vi "Facade.vi"(0 "Data In":T6, 2 "Display State In":T2={"Prompt"="Click to add", "Listbox"=refnum, "Required"={"Strings"=[], "Bottom"=FALSE, "Italic"=FALSE, "FG"=0, "BG"=0, "Bold"=FALSE}, "Items"=[], "Req'd"=[], "Events"={"Items Changed"=refnum, "List Changed"=refnum}, "Max Rows"=-1, "Default name"=""}, 3 "Container State":T5) -> (6 "Data Out":T6, 7 "Display State Out":T2={"Prompt"="Click to add", "Listbox"=refnum, "Required"={"Strings"=[], "Bottom"=FALSE, "Italic"=FALSE, "FG"=0, "BG"=0, "Bold"=FALSE}, "Items"=[], "Req'd"=[], "Events"={"Items Changed"=refnum, "List Changed"=refnum}, "Max Rows"=-1, "Default name"=""}, 8 "Action":T1)   [LabVIEW 2015, in "KListboxEx.xctl"]
uses:
  KListboxEx.xctl
  Data.ctl
  <vilib>/_xctls/Container State.ctl
  State.ctl
  Required.ctl
  Events.ctl
  Event Action.ctl
  <vilib>/_xctls/Action.ctl
  <vilib>/_xctls/XControlSupport.lvlib
panel:
  out "redisplay":bool
  out "drag from":i32
  in  "Listbox":i32(listbox)
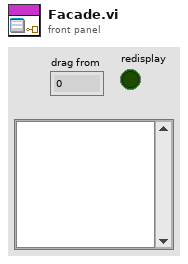
[diagram p1: front panel]
types:
  T1 = typedef "XControlSupport.lvlib/Action.ctl" = cluster{"Data Changed?":bool, "State Changed?":bool, "Action Name":string}
  T2 = typedef "KListboxEx.xctl/State.ctl" = cluster{"Prompt":string, "Listbox":refnum<vi>, "Required":T3, "Items":string[], "Req'd":bool[], "Events":T4, "Max Rows":i32, "Default name":string}
  T3 = typedef "KListboxEx.xctl/Required.ctl" = cluster{"Strings":string[], "Bottom":bool, "Italic":bool, "FG":u32, "BG":u32, "Bold":bool}
  T4 = typedef "KListboxEx.xctl/Events.ctl" = cluster{"Items Changed":refnum<user-event>, "List Changed":refnum<user-event>}
  T5 = typedef "XControlSupport.lvlib/Container State.ctl" = cluster{"Indicator?":bool, "Run Mode?":bool, " Refnum":refnum<vi>}
  T6 = typedef "KListboxEx.xctl/Data.ctl" = i32
  T7 = typedef "KListboxEx.xctl/Event Action.ctl" = enum16{"None", "Add", "Delete", "Move", "Edit", "Select"}
  T8 = typedef "LVPoint32TypeDef.ctl" = cluster{"Horizontal":i32, "Vertical":i32}
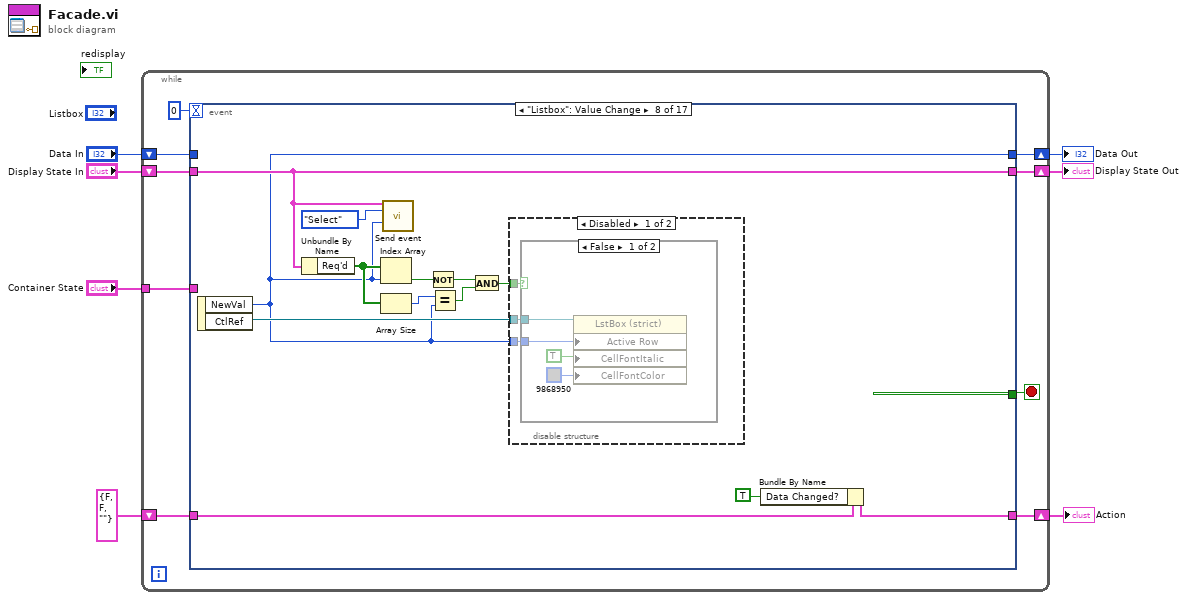
[diagram p0: block diagram]
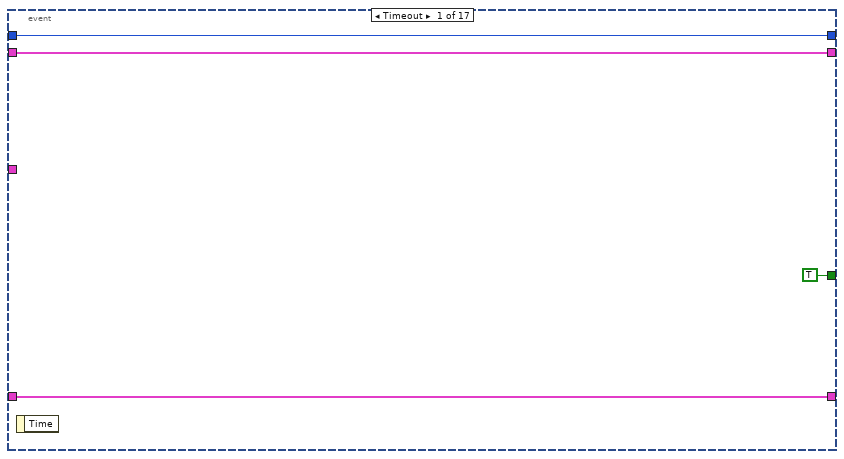
[diagram p2: hidden frame]
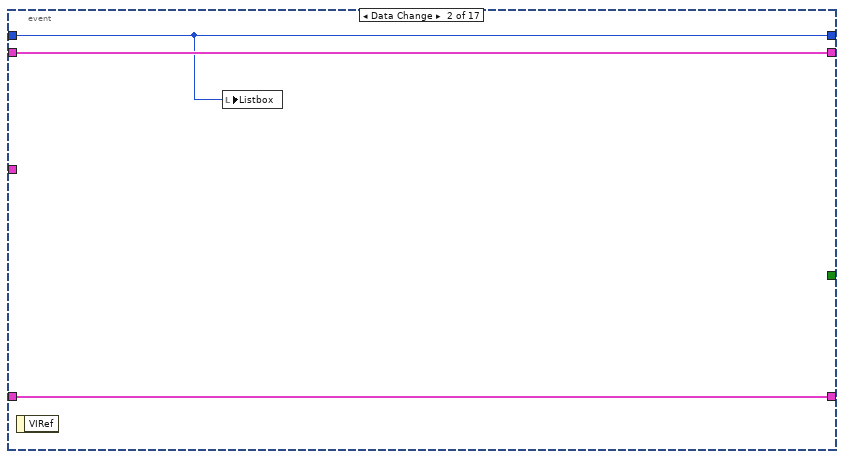
[diagram p3: hidden frame]
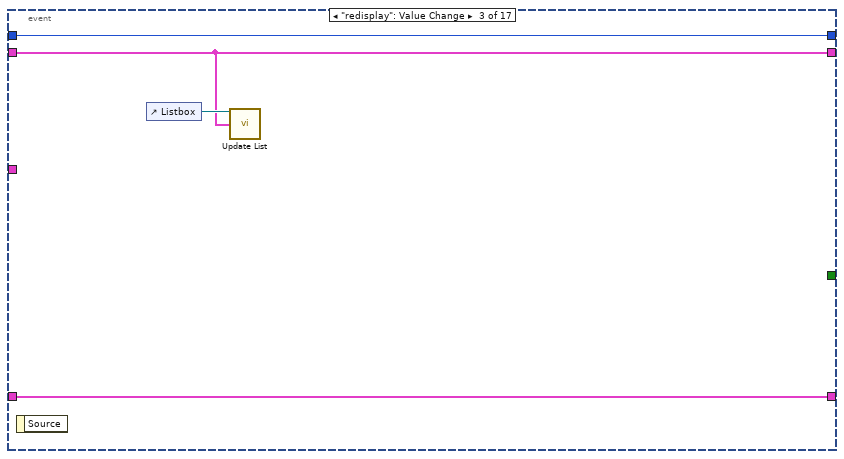
[diagram p4: hidden frame]
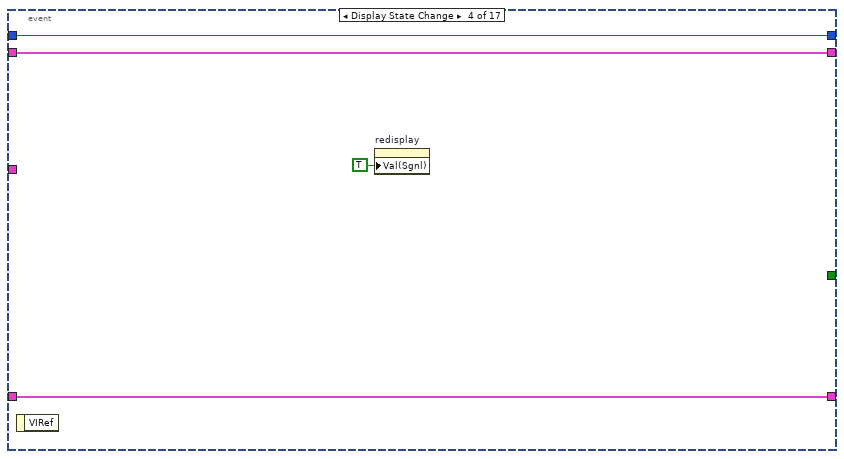
[diagram p5: hidden frame]
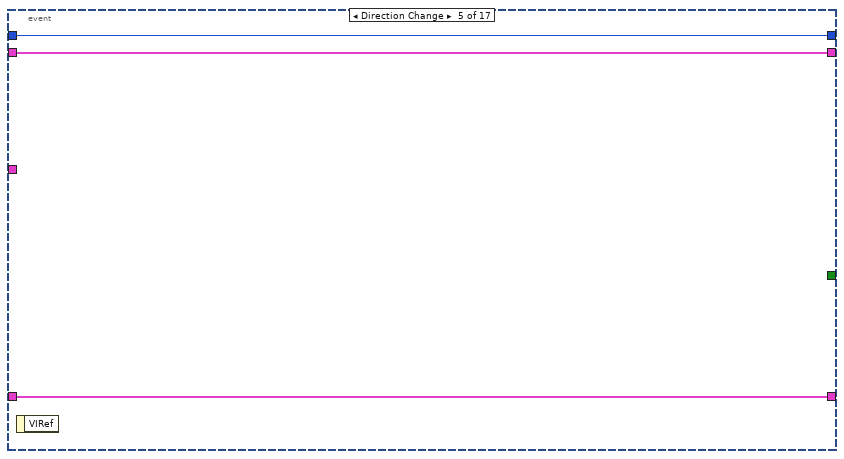
[diagram p6: hidden frame]
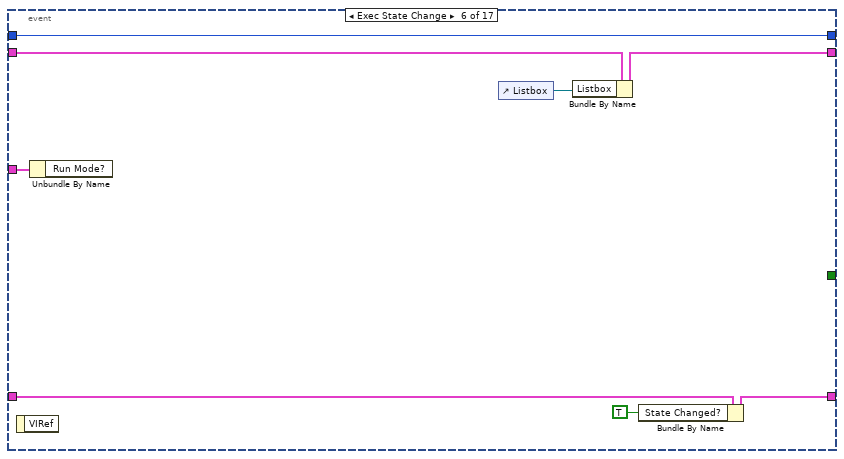
[diagram p7: hidden frame]
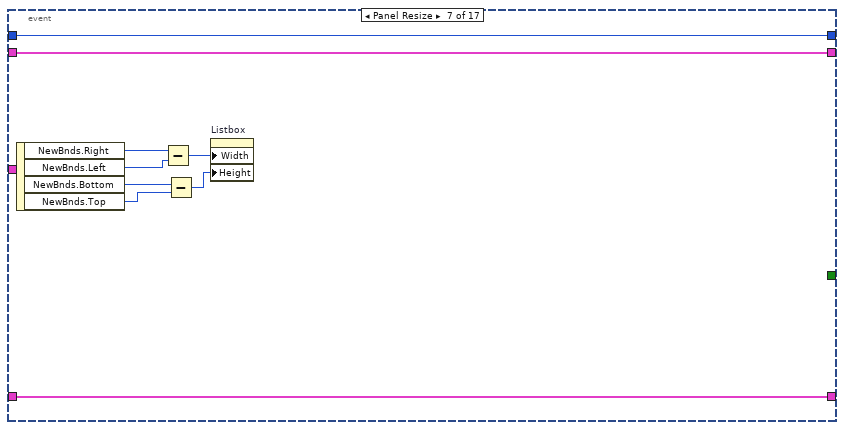
[diagram p8: hidden frame]
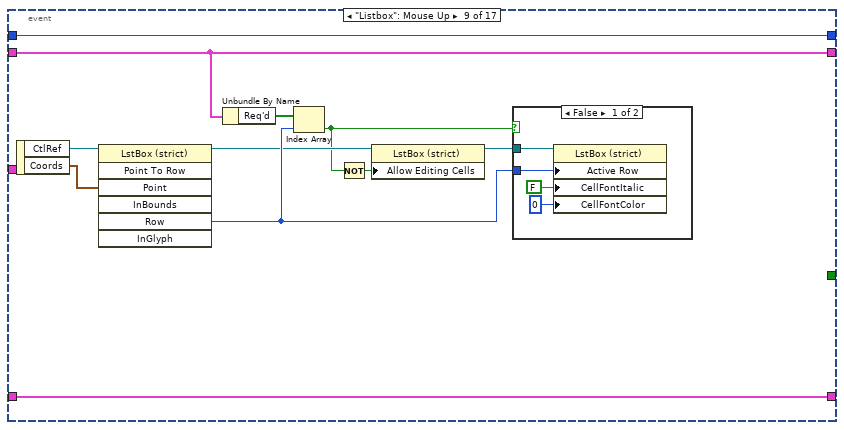
[diagram p11: hidden frame]
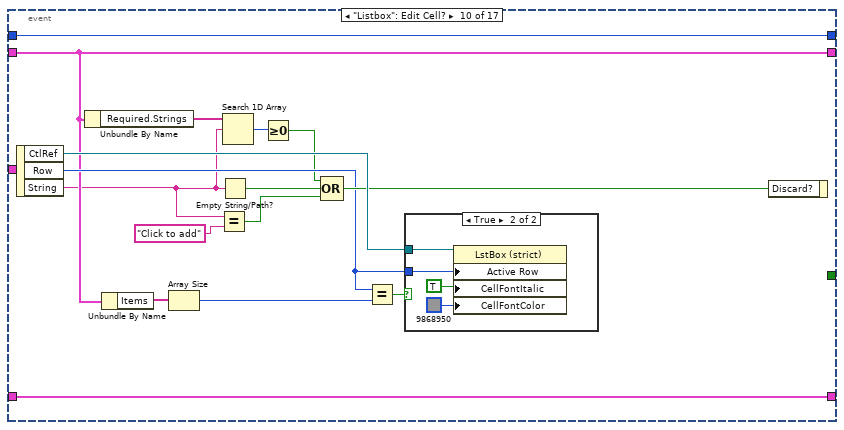
[diagram p13: hidden frame]
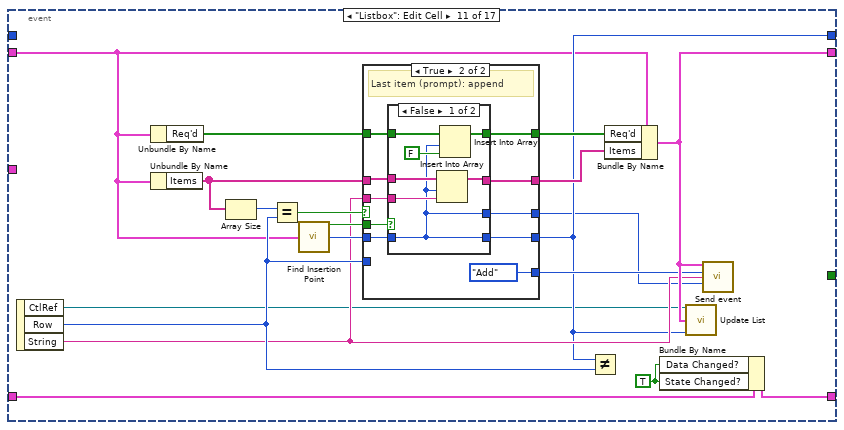
[diagram p15: hidden frame]
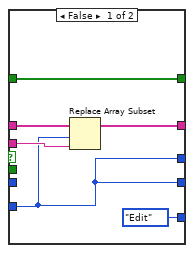
[diagram p16: hidden frame]
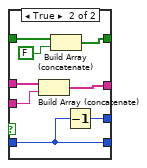
[diagram p17: hidden frame]
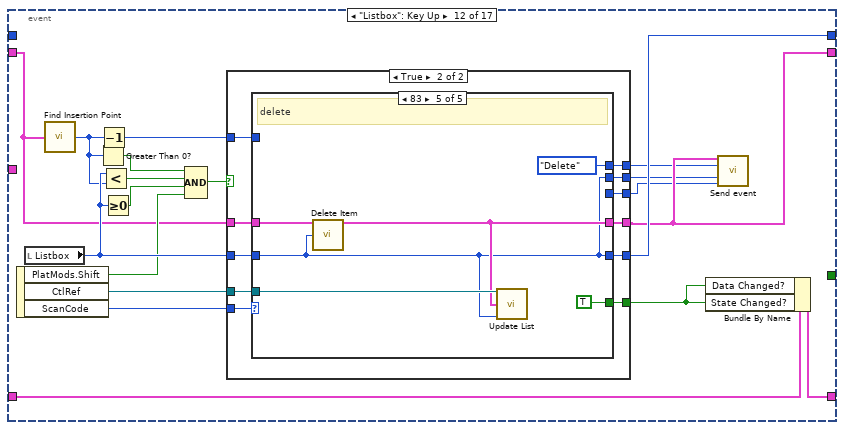
[diagram p18: hidden frame]
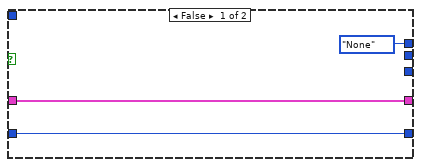
[diagram p19: hidden frame]
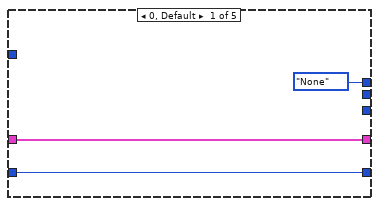
[diagram p20: hidden frame]
diagram:
  n1 = while {
    shift-right: [w15] -> w4
    shift-left: "Display State In" -> [w16]
    tunnel: "Container State" -> [w12]
    shift-right: [w10] -> w7
    shift-left: "Data In" -> [w11]
    shift-right: [w8] -> w2
    shift-left: T1 {"Data Changed?"=FALSE, "State Changed?"=FALSE, "Action Name"=""} ("Action") -> [w9]
    stop <- w14 stop-if-true
    n2 = event shown="[7] \"Listbox\": Value Change" {
      selector: _ -> [_ _ _ _ _ _ _ _ _ _ _ _ _ _ _ _ _]
      dyn-events: _ -> [_ _ _ _ _ _ _ _ _ _ _ _ _ _ _ _ _]
      timeout: 0 -> [_ _ _ _ _ _ _ _ _ _ _ _ _ _ _ _ _]
      tunnel: w16 -> [w18 w22 w24 w28 w34 w42 w51 w54 w77 w91 w108 w163 w249 w271 w273 w281 w284]
      tunnel: [w18 w22 w24 w28 w34 w39 w51 w54 w77 w91 w114 w161 w248 w271 w273 w281 w283] -> w15
      tunnel: [TRUE _ _ _ _ _ _ _ _ _ _ _ _ _ _ _ _] -> w14
      tunnel: w12 -> [_ _ _ _ _ w35 _ _ _ _ _ _ _ _ _ _ _]
      tunnel: w11 -> [w17 w21 w26 w31 w33 w41 w50 _ w82 w92 _ _ w252 w270 w274 w280 _]
      tunnel: [w17 w21 w26 w31 w33 w41 w50 w52 w82 w92 w111 w162 w252 w270 w274 w280 w286] -> w10
      tunnel: [w19 w23 w27 w30 w32 w37 w49 w63 w81 w102 w122 w174 w246 w269 w277 w279 w290] -> w8
      tunnel: w9 -> [w19 w23 w27 w30 w32 w40 w49 w64 w81 w102 w125 w175 w247 w269 w277 w279 w292]
      event Timeout {
        n3 = event-data() -> ()  [unwired: 1 in, 1 out]
      }
      event Data Change {
        n4 = event-data() -> ()  [unwired: 1 in, 1 out]
        n5 = local write "Listbox"(w21) -> ()
      }
      event "redisplay": Value Change {
        n6 = event-data() -> ()  [unwired: 1 in, 1 out]
        n7 = control-ref of="Listbox"() -> (w25:refnum<vi>)
        n8 = call "Update List.vi"("ListBox"=w25, "State"=w24) -> ()  [unwired: 13 in, 1 out]
      }
      event Display State Change {
        n9 = event-data() -> ()  [unwired: 1 in, 1 out]
        n10 = property on="redisplay" class="Bool (strict)"("Val(Sgnl)"=TRUE ("Value (Signaling)")) -> ()  [unwired: 2 in, 2 out]
      }
      event Direction Change {
        n11 = event-data() -> ()  [unwired: 1 in, 1 out]
      }
      event Exec State Change {
        n12 = event-data() -> ()  [unwired: 1 in, 1 out]
        n13 = Unbundle By Name(w35) -> ()  [unwired: 1 out]
        n14 = control-ref of="Listbox"() -> (w38:refnum<vi>)
        n15 = Bundle By Name(cluster=w42, "Listbox"=w38) -> (w39:T2)
        n16 = Bundle By Name(cluster=w40, "State Changed?"=TRUE) -> (w37:T1)
      }
      event Panel Resize {
        n17 = event-data() -> ("NewBnds.Right"=w48:i16, "NewBnds.Left"=w47:i16, "NewBnds.Bottom"=w46:i16, "NewBnds.Top"=w45:i16)  [unwired: 1 in]
        n18 = Subtract(x=w48, y=w47) -> (x-y=w44:i16)
        n19 = Subtract(x=w46, y=w45) -> (x-y=w43:i16)
        n20 = property on="Listbox" class="LstBox (strict)"("Width"=w44, "Height"=w43) -> ()  [unwired: 2 in, 2 out]
      }
      event "Listbox": Value Change {
        n21 = event-data() -> ("NewVal"=w52:i32, "CtlRef"=w60:refnum<vi>)  [unwired: 1 in]
        n22 = Unbundle By Name(w54) -> ("Req'd"=w59:bool[])
        n23 = Index Array(array=w59, index=w52) -> (element=w61:bool)
        n24 = Array Size(array=w59) -> (size(s)=w58:i32)
        n25 = call "Send event.vi"("State"=w54, "Action"=Event_Action."Select", "Start row"=w52) -> ()  [unwired: 13 in]
        n26 = Not(x=w61) -> (.not. x?=w55:bool)
        n27 = Equal?(x=w58, y=w52) -> (x = y?=w56:bool)
        n28 = And(x=w55, y=w56) -> (x .and. y?=w57:bool)
        n29 = disable-structure shown="Disabled" {
          disable-tunnel: w60 -> [w67 _]
          disable-tunnel: w52 -> [w66 _]
          disable-tunnel: w57 -> [w65 _]
          frame Disabled {
            n30 = case shown="False" w65 {
              tunnel: w67 -> [w69 _]
              tunnel: w66 -> [w68 _]
              frame False {
                n31 = property on="Property Node" class="LstBox (strict)"(reference=w69, "Active Row"=w68, "CellFontItalic"=TRUE ("Active Cell:Cell Font:Italic"), "CellFontColor"=u32 9868950) -> ()  [unwired: 1 in, 2 out]
              }
              frame True {
              }
            }
          }
          frame Enabled {
          }
        }
        n32 = Bundle By Name(cluster=w64, "Data Changed?"=TRUE) -> (w63:T1)
      }
      event "Listbox": Mouse Up {
        n33 = event-data() -> ("CtlRef"=w80:refnum<vi>, "Coords"=w79:T8)  [unwired: 1 in]
        n34 = invoke on="Invoke Node" class="LstBox (strict)" method="Point To Row"(reference=w80, "Point"=w79) -> (reference out=w75:refnum<vi>, "Row"=w78:i32)  [unwired: 5 in, 5 out]
        n35 = Unbundle By Name(w77) -> ("Req'd"=w76:bool[])
        n36 = Index Array(array=w76, index=w78) -> (element=w72:bool)
        n37 = Not(x=w72) -> (.not. x?=w73:bool)
        n38 = property class="LstBox (strict)"(reference=w75, "Allow Editing Cells"=w73) -> (reference out=w74:refnum<vi>)  [unwired: 1 in, 1 out]
        n39 = case shown="False" w72 {
          tunnel: w78 -> [w84 _]
          tunnel: w74 -> [w83 _]
          frame False {
            n40 = property on="Property Node" class="LstBox (strict)"(reference=w83, "Active Row"=w84, "CellFontItalic"=FALSE ("Active Cell:Cell Font:Italic"), "CellFontColor"=u32 0 ("Active Cell:Cell Font:Color")) -> ()  [unwired: 1 in, 2 out]
          }
          frame True {
          }
        }
      }
      event "Listbox": Edit Cell? {
        n41 = event-data() -> ("CtlRef"=w98:refnum<vi>, "Row"=w96:i32, "String"=w89:string)  [unwired: 1 in]
        n42 = Unbundle By Name(w91) -> ("Required.Strings"=w90:string[])
        n43 = Unbundle By Name(w91) -> ("Items"=w93:string[])
        n44 = Array Size(array=w93) -> (size(s)=w95:i32)
        n45 = Equal?(x=w89, y="Click to add" ("x")) -> (x = y?=w99:bool)
        n46 = Empty String/Path?(string/path=w89) -> (empty?=w100:bool)
        n47 = Search 1D Array(1D array=w90, element=w89) -> (index of element=w88:i32)  [unwired: 1 in]
        n48 = Greater Or Equal To 0?(x=w88) -> (x >= 0?=w87:bool)
        n49 = Compound Arithmetic op=OR(w87, w100, w99) -> (w97:bool)
        n50 = Equal?(x=w96, y=w95) -> (x = y?=w94:bool)
        n51 = case shown="True" w94 {
          tunnel: w98 -> [_ w105]
          tunnel: w96 -> [_ w104]
          frame False {
          }
          frame True {
            n52 = property on="Property Node" class="LstBox (strict)"(reference=w105, "Active Row"=w104, "CellFontItalic"=TRUE ("Active Cell:Cell Font:Italic"), "CellFontColor"=u32 9868950) -> ()  [unwired: 1 in, 2 out]
          }
        }
        n53 = event-data("Discard?"=w97) -> ()  [unwired: 1 in, 1 out]
      }
      event "Listbox": Edit Cell {
        w107 = TRUE ("Data Changed?")
        n54 = event-data() -> ("CtlRef"=w110:refnum<vi>, "Row"=w117:i32, "String"=w113:string)  [unwired: 1 in]
        n55 = Unbundle By Name(w108) -> ("Req'd"=w120:bool[])
        n56 = Unbundle By Name(w108) -> ("Items"=w121:string[])
        n57 = Array Size(array=w121) -> (size(s)=w124:i32)
        n58 = Equal?(x=w124, y=w117) -> (x = y?=w123:bool)
        n59 = call "Find Insertion Point.vi"("State"=w108) -> ("Append"=w118:bool, "Insert at"=w116:i32)  [unwired: 13 in]
        n60 = case shown="True" w123 {
          tunnel: w113 -> [w130 w141]
          tunnel: [w131 w140] -> w115
          tunnel: w121 -> [w129 w139]
          tunnel: w120 -> [w128 w138]
          tunnel: [w128 w137] -> w119
          tunnel: w118 -> [_ w136]
          tunnel: w117 -> [w126 _]
          tunnel: w116 -> [_ w135]
          tunnel: [w126 w134] -> w111
          tunnel: [Event_Action."Edit" ("Action") Event_Action."Add" ("Action")] -> w112
          tunnel: [w126 w132] -> w109
          frame False {
            n61 = Replace Array Subset(array=w129, new element=w130, index=w126) -> (w131:string[])
          }
          frame True {
            # "Last item (prompt): append"
            n62 = case shown="False" w136 {
              tunnel: w141 -> [w143 w156]
              tunnel: [w144 w155] -> w140
              tunnel: w139 -> [w145 w154]
              tunnel: w138 -> [w148 w153]
              tunnel: [w147 w152] -> w137
              tunnel: w135 -> [w142 w150]
              tunnel: [w142 w150] -> w134
              tunnel: [w142 w149] -> w132
              frame False {
                n63 = Insert Into Array(array=w145, index=w142, new element=w143) -> (w144:string[])
                n64 = Insert Into Array(array=w148, index=w142, new element=FALSE ("new element/subarray")) -> (w147:bool[])
              }
              frame True {
                n65 = Build Array (concatenate)(w154, w156) -> (w155:string[])
                n66 = Build Array (concatenate)(w153, FALSE) -> (w152:bool[])
                n67 = Decrement(x=w150) -> (x-1=w149:i32)
              }
            }
          }
        }
        n68 = Not Equal?(x=w111, y=w117) -> ()  [unwired: 1 out]
        n69 = Bundle By Name(cluster=w108, "Req'd"=w119, "Items"=w115) -> (w114:T2)
        n70 = Bundle By Name(cluster=w125, "Data Changed?"=w107, "State Changed?"=w107) -> (w122:T1)
        n71 = call "Update List.vi"("ListBox"=w110, "State"=w114, "Row"=w111) -> ()  [unwired: 12 in, 1 out]
        n72 = call "Send event.vi"("State"=w114, "Action"=w112, "Name"=w113, "Start row"=w109) -> ()  [unwired: 12 in]
      }
      event "Listbox": Key Up {
        n73 = event-data() -> ("PlatMods.Shift"=w167:bool, "CtlRef"=w168:refnum<vi>, "ScanCode"=w169:i16)  [unwired: 1 in]
        n74 = local read "Listbox"() -> (w170:i32)
        n75 = call "Find Insertion Point.vi"("State"=w163) -> ("Insert at"=w164:i32)  [unwired: 13 in, 1 out]
        n76 = Greater Than 0?(x=w164) -> (x > 0?=w172:bool)
        n77 = Decrement(x=w164) -> (x-1=w165:i32)
        n78 = Less?(x=w170, y=w164) -> (x < y?=w166:bool)
        n79 = Greater Or Equal To 0?(x=w170) -> (x >= 0?=w173:bool)
        n80 = Compound Arithmetic op=AND(w172, w166, w173, w167) -> (w171:bool)
        n81 = case shown="True" w171 {
          tunnel: w169 -> [_ w189]
          tunnel: w163 -> [w178 w188]
          tunnel: w170 -> [w177 w187]
          tunnel: [w178 w186] -> w161
          tunnel: [_ w185] -> w160
          tunnel: w168 -> [_ w184]
          tunnel: w165 -> [_ w183]
          tunnel: [w177 w182] -> w162
          tunnel: [Event_Action."None" ("Action") w179] -> w159
          tunnel: [_ w181] -> w158
          tunnel: [_ w180] -> w157
          frame False {
          }
          frame True {
            n82 = case shown="83" w189 {
              tunnel: w188 -> [w192 w202 w217 w237 w243]
              tunnel: w187 -> [w191 w198 w219 w232 w239]
              tunnel: [w192 w197 w216 w234 w241] -> w186
              tunnel: [_ w201 w222 TRUE TRUE] -> w185
              tunnel: w184 -> [_ w200 w221 w235 w242]
              tunnel: w183 -> [_ _ w218 _ _]
              tunnel: [w191 w196 w215 w232 w239] -> w182
              tunnel: [_ w195 w213 w232 w239] -> w181
              tunnel: [_ w194 w212 _ _] -> w180
              tunnel: [Event_Action."None" ("Action") w193 w214 Event_Action."Add" ("Action") Event_Action."Delete" ("Action")] -> w179
              frame 0, Default {
              }
              frame 72 {
                # "up arrow"
                n83 = Greater Than 0?(x=w198) -> (x > 0?=w199:bool)
                n84 = case shown="True" w199 {
                  tunnel: w202 -> [w204 w210]
                  tunnel: [_ TRUE] -> w201
                  tunnel: w200 -> [_ w209]
                  tunnel: w198 -> [w203 w207]
                  tunnel: [w204 w208] -> w197
                  tunnel: [w203 w206] -> w196
                  tunnel: [_ w207] -> w195
                  tunnel: [_ w206] -> w194
                  tunnel: [_ Event_Action."Move" ("Action")] -> w193
                  frame False {
                  }
                  frame True {
                    n85 = Decrement(x=w207) -> (x-1=w206:i32)
                    n86 = call "Move Item.vi"("Display State In"=w210, "Move from"=w207, "Move to"=w206) -> ("Display State Out"=w208:T2)  [unwired: 12 in]
                    n87 = call "Update List.vi"("ListBox"=w209, "State"=w208, "Row"=w206) -> ()  [unwired: 12 in, 1 out]
                  }
                }
              }
              frame 80 {
                # "down arrow"
                n88 = Less?(x=w219, y=w218) -> (x < y?=w220:bool)
                n89 = case shown="True" w220 {
                  tunnel: [_ TRUE] -> w222
                  tunnel: w221 -> [_ w229]
                  tunnel: w219 -> [w223 w226]
                  tunnel: w217 -> [w224 w230]
                  tunnel: [w224 w228] -> w216
                  tunnel: [w223 w225] -> w215
                  tunnel: [_ Event_Action."Move" ("Action")] -> w214
                  tunnel: [_ w226] -> w213
                  tunnel: [_ w225] -> w212
                  frame False {
                  }
                  frame True {
                    n90 = Increment(x=w226) -> (x+1=w225:i32)
                    n91 = call "Move Item.vi"("Display State In"=w230, "Move from"=w226, "Move to"=w225) -> ("Display State Out"=w228:T2)  [unwired: 12 in]
                    n92 = call "Update List.vi"("ListBox"=w229, "State"=w228, "Row"=w225) -> ()  [unwired: 12 in, 1 out]
                  }
                }
              }
              frame 82 {
                # "insert"
                n93 = call "Insert Item.vi"("State In"=w237, "Insert at"=w232) -> ("State Out"=w234:T2)  [unwired: 13 in]
                n94 = call "Update List.vi"("ListBox"=w235, "State"=w234, "Row"=w232) -> ("reference out"=w236:refnum<vi>)  [unwired: 12 in]
                n95 = property class="LstBox (strict)"(reference=w236, "EditRow"=w232) -> ()  [unwired: 1 in, 2 out]
              }
              frame 83 {
                # "delete"
                n96 = call "Delete Item.vi"("State In"=w243, "Delete at"=w239) -> ("State Out"=w241:T2)  [unwired: 13 in]
                n97 = call "Update List.vi"("ListBox"=w242, "State"=w241, "Row"=w239) -> ()  [unwired: 12 in, 1 out]
              }
            }
          }
        }
        n98 = Bundle By Name(cluster=w175, "Data Changed?"=w160, "State Changed?"=w160) -> (w174:T1)
        n99 = call "Send event.vi"("State"=w161, "Action"=w159, "Start row"=w158, "End row"=w157) -> ()  [unwired: 12 in]
      }
      event "Listbox": Shortcut Menu Selection (User) {
        n100 = event-data() -> ("ItemTag"=w251:string, "CtlRef"=w245:refnum<vi>)  [unwired: 1 in]
        n101 = local read "Listbox"() -> (w250:i32)
        n102 = case shown="\"cmDelete\"" w251 {
          tunnel: w250 -> [_ w255]
          tunnel: w249 -> [w254 w262]
          tunnel: [w254 w256] -> w248
          tunnel: w247 -> [w253 w260]
          tunnel: [w253 w259] -> w246
          tunnel: w245 -> [_ w257]
          frame "", Default {
          }
          frame "cmDelete" {
            w258 = TRUE
            n103 = call "Delete Item.vi"("State In"=w262, "Delete at"=w255) -> ("State Out"=w256:T2)  [unwired: 13 in]
            n104 = call "Update List.vi"("ListBox"=w257, "State"=w256, "Row"=w255) -> ()  [unwired: 12 in, 1 out]
            n105 = call "Send event.vi"("State"=w256, "Action"=Event_Action."Delete", "Start row"=w255) -> ()  [unwired: 13 in]
            n106 = Bundle By Name(cluster=w260, "Data Changed?"=w258, "State Changed?"=w258) -> (w259:T1)
          }
        }
      }
      event "Listbox": Key Down? {
        n107 = event-data() -> ("PlatMods.Shift"=w268:bool, "ScanCode"=w266:i16)  [unwired: 1 in]
        n108 = Search 1D Array(1D array=i16[] [72, 80], element=w266) -> (index of element=w265:i32)  [unwired: 1 in]
        n109 = Greater Or Equal To 0?(x=w265) -> (x >= 0?=w264:bool)
        n110 = And(x=w268, y=w264) -> (x .and. y?=w267:bool)
        n111 = event-data("Discard?"=w267) -> ()  [unwired: 1 in, 1 out]
      }
      event "Listbox": Drag Starting? {
        n112 = event-data() -> ()  [unwired: 1 in, 1 out]
        n113 = local read "Listbox"() -> (w276:i32)
        n114 = call "Find Insertion Point.vi"("State"=w273) -> ("Insert at"=w272:i32)  [unwired: 13 in, 1 out]
        n115 = Greater Or Equal?(x=w276, y=w272) -> (x >= y?=w275:bool)
        n116 = event-data("Discard?"=w275) -> ()  [unwired: 1 in, 1 out]
      }
      event "Listbox": Drag Starting {
        n117 = event-data() -> ()  [unwired: 1 in, 1 out]
        n118 = local read "Listbox"() -> (→"drag from":i32)
      }
      event "Listbox": Drag Ended {
        n119 = event-data() -> ("CtlRef"=w288:refnum<vi>, "Result"=w291:enum16{"Drop Cancel", "Drop Move", "Drop Copy"})  [unwired: 1 in]
        n120 = local read "Listbox"() -> (w285:i32)
        n121 = call "Find Insertion Point.vi"("State"=w284) -> ("Insert at"=w287:i32)  [unwired: 13 in, 1 out]
        n122 = local read "drag from"() -> (w289:i32)
        n123 = case shown="\"Drop Move\"" w291 {
          tunnel: w284 -> [w294 w299]
          tunnel: [w294 w298] -> w283
          tunnel: [_ TRUE] -> w282
          tunnel: w289 -> [_ w296]
          tunnel: w285 -> [w293 w303]
          tunnel: w288 -> [_ w301]
          tunnel: w287 -> [_ w300]
          tunnel: [w293 w295] -> w286
          frame "Drop Cancel", Default {
          }
          frame "Drop Move" {
            n124 = Decrement(x=w300) -> (x-1=w302:i32)
            n125 = Max & Min(x=w303, y=w302) -> (min(x,y)=w295:i32)  [unwired: 1 out]
            n126 = call "Move Item.vi"("Display State In"=w299, "Move from"=w296, "Move to"=w295) -> ("Display State Out"=w298:T2)  [unwired: 12 in]
            n127 = call "Update List.vi"("ListBox"=w301, "State"=w298, "Row"=w295) -> ()  [unwired: 12 in, 1 out]
            n128 = call "Send event.vi"("State"=w298, "Action"=Event_Action."Move", "Start row"=w296, "End row"=w295) -> ()  [unwired: 12 in]
          }
        }
        n129 = Bundle By Name(cluster=w292, "Data Changed?"=w282, "State Changed?"=w282) -> (w290:T1)
      }
    }
  }
  "Display State Out" <- w4
  "Data Out" <- w7
  "Action" <- w2
